vi "change lcr voltage.vi"(10 "voltage":dbl, 11 "lcr in":refnum<visa-resource-name>) -> (3 "lcr out":refnum<visa-resource-name>)   [LabVIEW 2018]
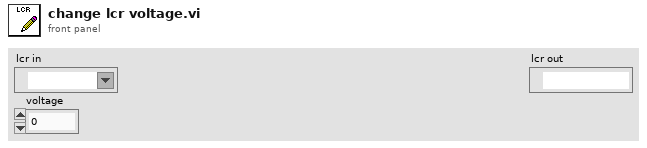
[diagram p1: front panel]
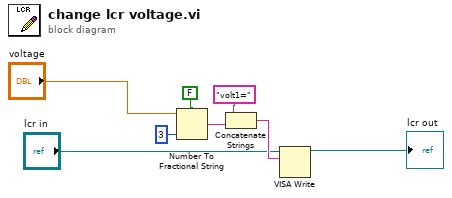
[diagram p0: block diagram]
diagram:
  n1 = Number To Fractional String(use system decimal point (T)=FALSE, number="voltage", precision (6)=i16 3) -> (F-format string=w6:string)  [unwired: 1 in]
  n2 = Concatenate Strings("volt1=" ("string"), w6) -> (w4:string)
  n3 = VISA Write(VISA resource name="lcr in", write buffer=w4) -> (VISA resource name out=→"lcr out":refnum<visa-resource-name>)  [unwired: 1 in, 2 out]
